vi "ЗНАЧЕНИЕ НЕКОР.vi"() -> ()   [LabVIEW 2016, in "Library.lvlib"]
uses:
  Granule-2000AT/PC/llb/Library.lvlib
panel:
  in  "OK Button":bool
  out "?":string
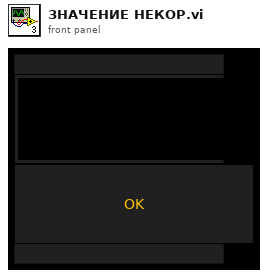
[diagram p1: front panel]
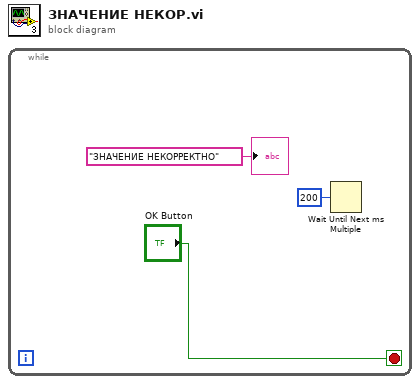
[diagram p0: block diagram]
diagram:
  n1 = while {
    stop <- "OK Button" stop-if-true
    n2 = Wait Until Next ms Multiple(millisecond multiple=u32 200) -> ()  [unwired: 1 out]
    "?" <- "ЗНАЧЕНИЕ НЕКОРРЕКТНО" ("String")
  }
